vi "FPServerSetData.vi"(0 "Page":string, 2 "Data":string[][](array[string]), 5 "error in (no error)":errorcluster) -> (19 "error out":errorcluster)   [LabVIEW 2014, in "FrontPanelPublisher.lvlib" / "FrontPanelManager.lvclass"]
uses:
  FrontPanelManager.lvclass
  protected/FPServerMessage.ctl
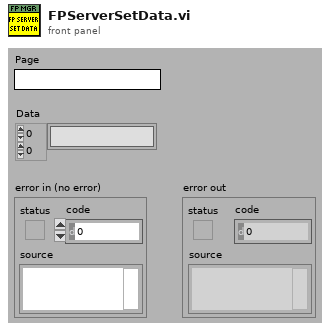
[diagram p1: front panel]
types:
  T1 = typedef "FrontPanelPublisher.lvlib/FrontPanelManager.lvclass/FPServerMessage.ctl" = cluster{"Message":string, "Page":string, "Data":string[][], "Connection ID":u64}
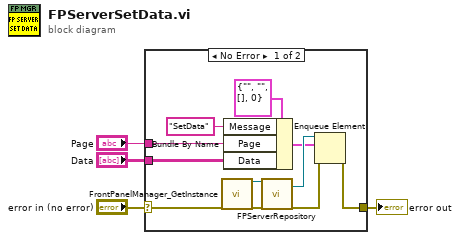
[diagram p0: block diagram]
diagram:
  n1 = case shown="No Error" "error in (no error)" {
    selector: "error in (no error)" -> [w12 w16]
    tunnel: [w5 w16] -> w3
    tunnel: "Page" -> [w7 _]
    tunnel: "Data" -> [w6 _]
    frame No Error {
      n2 = call "FrontPanelManager_GetInstance.vi"("error in (no error)"=w12) -> ("reference out"=w13:refnum<class "FrontPanelManager.lvclass">, "error out"=w11:errorcluster)  [unwired: 14 in, 3 out]
      n3 = Bundle By Name(cluster=T1 {"Message"="", "Page"="", "Data"=[], "Connection ID"=0} ("element"), "Message"="SetData", "Page"=w7, "Data"=w6) -> (w9:T1)
      n4 = call "FPServerRepository.vi"("reference in"=w13, "error in (no error)"=w11) -> ("ToProcessQueue"=w10:refnum<queue>, "error out"=w14:errorcluster)  [unwired: 11 in, 5 out]
      n5 = Enqueue Element(queue=w10, element=w9, error in (no error)=w14) -> (error out=w5:errorcluster)  [unwired: 1 in, 2 out]
    }
    frame Error {
    }
  }
  "error out" <- w3
